vi "UTIL_Send Close to Error Queue v1_0_0.vi"(8 "error in (no error)":errorcluster, 11 "name (Error)":string="Error") -> (0 "error out":errorcluster)   [LabVIEW 2015]
doc: "UTIL_Send Close to Error Queue v1_0_0.vi\n\nThis vi Sends a close command to the Error Q.vi. It will cause the Error Q.vi to put a note in the error log with a current time stamp stating that the error logging was stopped.\n\nthe Error Q.vi will respond to this command by shutting itself down when called.\n\nNote: if the Error Q.vi is not running this will prompt the user with an error.\n\nCreated 2006 by\n\nJ. Daren Suntych\nNational Analytics\n970-397-0764"
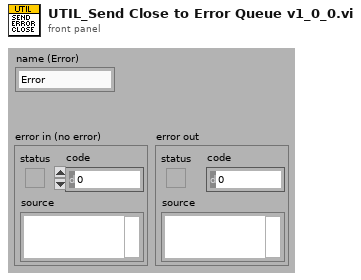
[diagram p1: front panel]
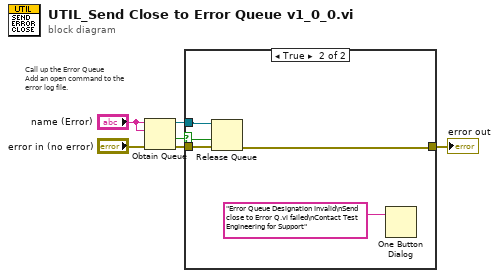
[diagram p0: block diagram]
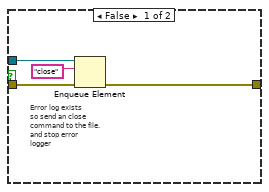
[diagram p2: hidden frame]
diagram:
  # "Call up the Error Queue\nAdd an open command to the \nerror log file."
  n1 = Obtain Queue(name (unnamed)="name (Error)", element data type="name (Error)", error in (no error)="error in (no error)") -> (queue out=w4:refnum<queue>, created new?=w2:bool, error out=w3:errorcluster)  [unwired: 2 in]
  n2 = case shown="True" w2 {
    selector: w2 -> [_ w13]
    tunnel: w4 -> [w10 w15]
    tunnel: w3 -> [w9 w14]
    tunnel: [w8 w12] -> w1
    frame False {
      # "Error log exists \nso send an close \ncommand to the file.\nand stop error\nlogger"
      n3 = Enqueue Element(queue=w10, element="close" ("queue element"), error in (no error)=w9) -> (error out=w8:errorcluster)  [unwired: 3 out]
    }
    frame True {
      n4 = Release Queue(queue=w15, force destroy? (F)=w13, error in (no error)=w14) -> (error out=w12:errorcluster)  [unwired: 2 out]
      n5 = One Button Dialog(message="Error Queue Designation Invalid\nSend close to Error Q.vi failed\nContact Test Engineering for Support" ("window title (\"\")")) -> ()  [unwired: 2 out]
    }
  }
  "error out" <- w1
